vi "line_save.vi"(7 "double? (F)":bool, 8 "error in (no error)":errorcluster, 9 "save type":T1, 10 "index":i32, 11 "AnalysisRAPS in":refnum<class "AnalysisRAPS.lvclass">) -> (0 "error out":errorcluster, 3 "AnalysisRAPS out":refnum<class "AnalysisRAPS.lvclass">)   [LabVIEW 2010, in "AnalysisRAPS.lvclass"]
uses:
  AnalysisRAPS.lvclass
  saving_type.ctl
  AnalysisRAPS.lvclass/AnalysisRAPS.ctl
  <vilib>/Utility/file.llb/Write To Spreadsheet File (DBL).vi
  <vilib>/Utility/file.llb/Write To Spreadsheet File (I64).vi
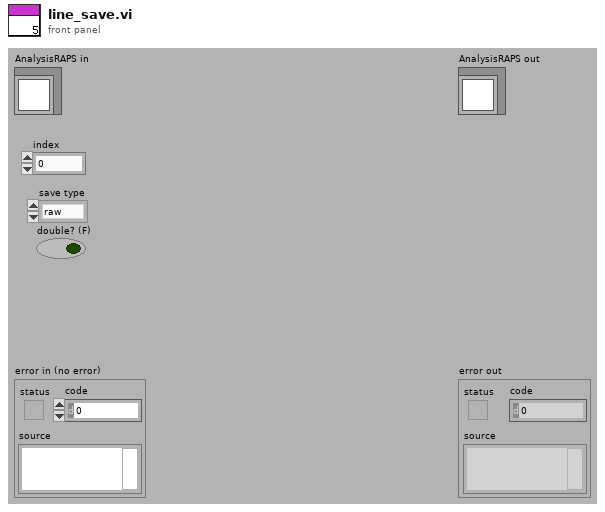
[diagram p1: front panel]
types:
  T1 = typedef "AnalysisRAPS.lvclass/saving_type.ctl" = enum16{"raw", "average"}
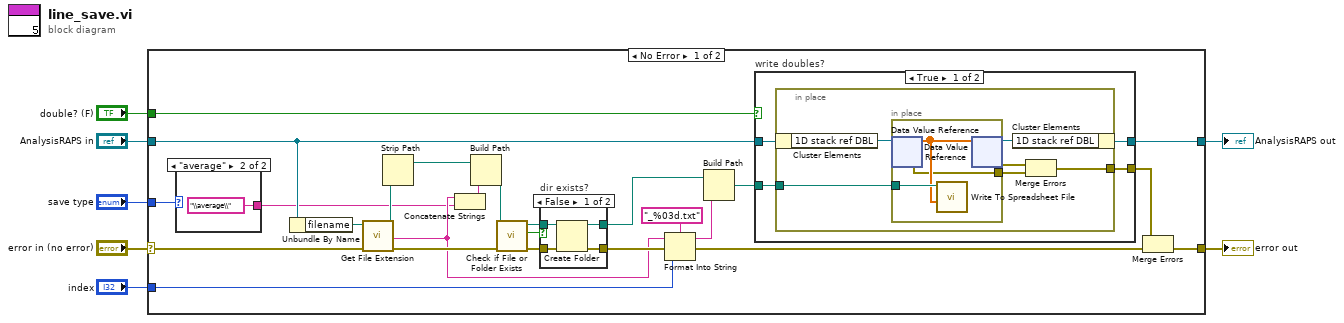
[diagram p0: block diagram]
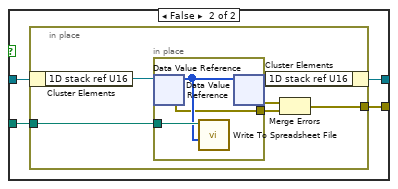
[diagram p2: hidden frame]
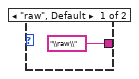
[diagram p3: hidden frame]
diagram:
  n1 = case shown="No Error" "error in (no error)" {
    selector: "error in (no error)" -> [w30 w68]
    tunnel: [w21 w68] -> w6
    tunnel: [w32 w67] -> w4
    tunnel: "AnalysisRAPS in" -> [w31 w67]
    tunnel: "index" -> [w25 _]
    tunnel: "save type" -> [w10 _]
    tunnel: "double? (F)" -> [w8 _]
    frame No Error {
      n2 = case shown="\"average\"" w10 {
        tunnel: ["\\raw\\" ("string") "\\average\\" ("string")] -> w9
        frame "raw", Default {
        }
        frame "average" {
        }
      }
      n3 = Unbundle By Name(w31) -> ("filename"=w29:path)
      n4 = call <vilib>:"Get File Extension.vi"("error in (no error)"=w30, "file"=w29) -> ("error out"=w14:errorcluster, "filename without extension"=w12:string, "dup file"=w28:path)  [unwired: 6 in, 1 out]
      n5 = Strip Path(path=w28) -> (stripped path=w20:path)  [unwired: 1 out]
      n6 = Concatenate Strings(w12, w9) -> (w17:string)
      n7 = Build Path(base path=w20, name or relative path=w17) -> (appended path=w16:path)
      n8 = call <vilib>:"Check if File or Folder Exists.vi"("error in (no error)"=w14, "path"=w16) -> ("error out"=w13:errorcluster, "file or folder exists?"=w11:bool, "dup path"=w15:path)  [unwired: 7 in]
      n9 = case "dir exists?" shown="False" w11 {
        tunnel: [w64 w66] -> w19
        tunnel: [w63 w65] -> w18
        tunnel: w15 -> [w62 w66]
        tunnel: w13 -> [w61 w65]
        frame False {
          n10 = Create Folder(path (use dialog)=w62, error in=w61) -> (created path=w64:path, error out=w63:errorcluster)  [unwired: 1 in, 1 out]
        }
        frame True {
        }
      }
      n11 = Format Into String(format string="_%03d.txt", initial string=w12, error in=w18, w25) -> (resulting string=w27:string, error out=w22:errorcluster)
      n12 = Build Path(base path=w19, name or relative path=w27) -> (appended path=w26:path)
      n13 = case "write doubles?" shown="True" w8 {
        tunnel: [w36 w49] -> w32
        tunnel: w31 -> [w35 w48]
        tunnel: w26 -> [w34 w47]
        tunnel: [w33 w46] -> w23
        frame True {
          n14 = in-place {
            in-place-border: w34 -> [w40]
            in-place-border: [w37] -> w33
            n15 = in-place-cluster #1(w35) -> ("1D stack ref DBL"=w42:refnum<data-value>)
            n16 = in-place {
              in-place-border: w40 -> [w45]
              in-place-border: [w43] -> w38
              n17 = in-place-dvr #2(w42) -> (w44:dbl[], w43:errorcluster)
              n18 = call-poly <vilib>:"Write To Spreadsheet File.vi"("1D data"=w44, "file path (dialog if empty)"=w45) -> ()  [unwired: 6 in, 1 out]
              n19 = in-place-dvr #2(w44) -> (w41:refnum<data-value>, w39:errorcluster)
            }
            n20 = in-place-cluster #1("1D stack ref DBL"=w41) -> (w36:refnum<class "AnalysisRAPS.lvclass">)
            n21 = Merge Errors(w39, w38) -> (w37:errorcluster)
          }
        }
        frame False {
          n22 = in-place {
            in-place-border: w47 -> [w53]
            in-place-border: [w50] -> w46
            n23 = in-place-cluster #3(w48) -> ("1D stack ref U16"=w55:refnum<data-value>)
            n24 = in-place {
              in-place-border: w53 -> [w58]
              in-place-border: [w56] -> w51
              n25 = in-place-dvr #4(w55) -> (w57:u16[], w56:errorcluster)
              n26 = call-poly <vilib>:"Write To Spreadsheet File.vi"("1D data"=w57, "file path (dialog if empty)"=w58) -> ()  [unwired: 6 in, 1 out]
              n27 = in-place-dvr #4(w57) -> (w54:refnum<data-value>, w52:errorcluster)
            }
            n28 = in-place-cluster #3("1D stack ref U16"=w54) -> (w49:refnum<class "AnalysisRAPS.lvclass">)
            n29 = Merge Errors(w52, w51) -> (w50:errorcluster)
          }
        }
      }
      n30 = Merge Errors(w23, w22) -> (w21:errorcluster)
    }
    frame Error {
    }
  }
  "error out" <- w6
  "AnalysisRAPS out" <- w4
